vi "Read Measurement Interface.vi"(8 "error in (no error)":errorcluster, 11 "niRFSTS Sequence Flow in":refnum<class "niRFSTS Sequence Flow.lvclass">) -> (0 "error out":errorcluster, 2 "Measurement Interface.lvlibp:Measurement Interface":refnum<class "Measurement Interface.lvclass">, 3 "niRFSTS Sequence Flow out":refnum<class "niRFSTS Sequence Flow.lvclass">)   [LabVIEW 2018, in "niRFSTS Sequence Flow.lvclass"]
uses:
  niRFSTS Sequence Flow.lvclass
  Plugins/Measurement Interface.lvlibp/Measurement Interface.lvclass
  niRFSTS Sequence Flow.lvclass/niRFSTS Sequence Flow.ctl
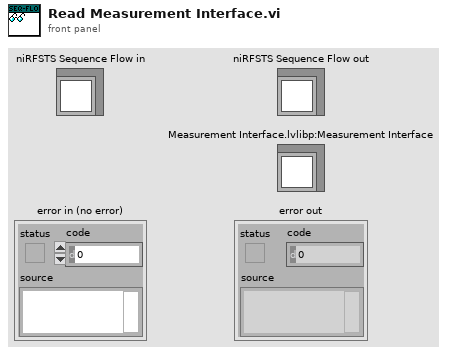
[diagram p1: front panel]
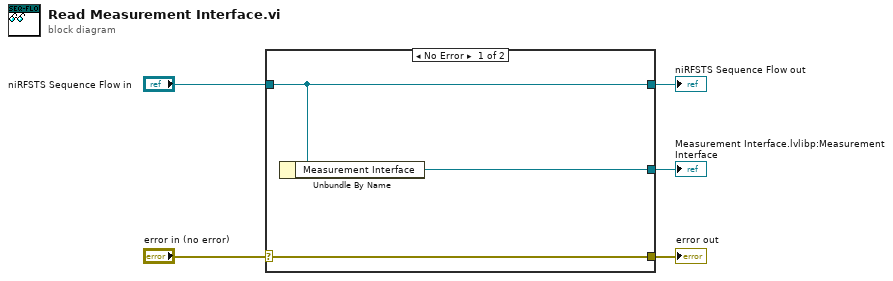
[diagram p0: block diagram]
diagram:
  n1 = case shown="No Error" "error in (no error)" {
    selector: "error in (no error)" -> [w8 w9]
    tunnel: [w8 w9] -> w4
    tunnel: [w7 w10] -> w2
    tunnel: "niRFSTS Sequence Flow in" -> [w7 w10]
    tunnel: [w6 _] -> w1
    frame No Error {
      n2 = Unbundle By Name(w7) -> ("Measurement Interface"=w6:refnum<class "Measurement Interface.lvclass">)
    }
    frame Error {
    }
  }
  "error out" <- w4
  "niRFSTS Sequence Flow out" <- w2
  "Measurement Interface.lvlibp:Measurement Interface" <- w1
